vi "P4CMD Close Project.vi"(8 "error in (no error)":errorcluster, 11 "source control reference in":T1) -> (0 "error out":errorcluster, 2 "status message":string)   [LabVIEW 2020, in "NI_SCC_P4CMD.lvlib"]
uses:
  <vilib>/SourceControl/Providers/P4CMD/NI_SCC_P4CMD.lvlib
  <vilib>/SourceControl/sccapi/SCCAPI Refnum.ctl
  <vilib>/SourceControl/Providers/P4CMD/P4CMD Mgr Functions.ctl
  <vilib>/SourceControl/support/SCCSup Message Strings GLBL.vi
  <vilib>/SourceControl/sccapi/NI_SCC.lvlib
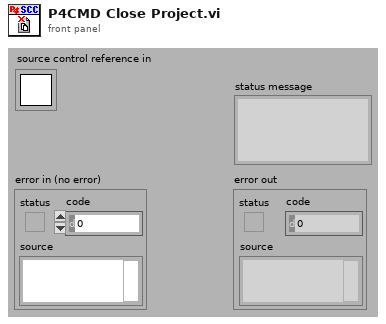
[diagram p1: front panel]
types:
  T1 = typedef "NI_SCC.lvlib/SCCAPI Refnum.ctl" = refnum<k1>
  T2 = typedef "NI_SCC_P4CMD.lvlib/P4CMD Mgr Functions.ctl" = enum16{"Init", "Open", "Set Config Opts", "Initialized?", "IsRefValid?", "Get Config Opts", "Get Global Commands", "Close", "Uninit"}
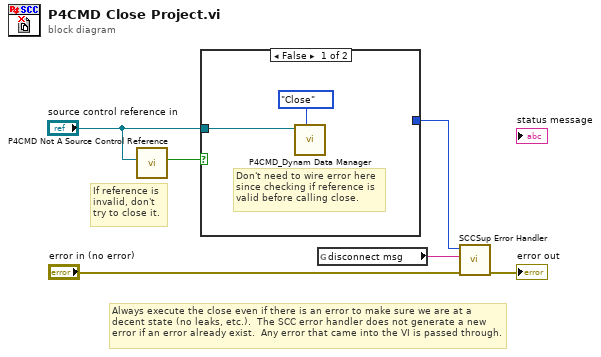
[diagram p0: block diagram]
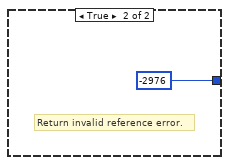
[diagram p2: hidden frame]
diagram:
  # "If reference is invalid, don't try to close it."
  # "Always execute the close even if there is an error to make sure we are at a decent state (no leaks, etc.).  The SCC error handler does not generate a new error if an error already exist.  Any error that came into the VI is passed through."
  n1 = call <vilib>:"P4CMD Not A Source Control Reference.vi"("source control reference in"="source control reference in") -> ("not a source control reference?"=w2:bool)  [unwired: 9 in, 1 out]
  n2 = case shown="False" w2 {
    tunnel: [_ -2976 ("result")] -> w6
    tunnel: "source control reference in" -> [w8 _]
    frame False {
      # "Don't need to wire error here since checking if reference is valid before calling close."
      n3 = call <vilib>:"P4CMD_Dynam Data Manager.vi"("function"=P4CMD_Mgr_Functions."Close", "source control reference in"=w8) -> ()  [unwired: 4 in, 6 out]
    }
    frame True {
      # "Return invalid reference error."
    }
  }
  n4 = global read "SCCSup Message Strings GLBL.vi" "disconnect msg"() -> (w4:string)
  n5 = call <vilib>:"SCCSup Error Handler.vi"("error in (no error)"="error in (no error)", "operation message"=w4, "scc error code"=w6) -> ("error out"=→"error out":errorcluster)  [unwired: 8 in]
